vi "USBGetBuffer.vi"() -> ()   [LabVIEW 2012]
uses:
  <vilib>/Instr/_visa.llb/VISA Open Access Mode.ctl
panel:
  out "read buffer 2":string
  out "string":string
  out "16bit integer 2":i16
  out "16bit integer":i16
  out "unsigned 16bit integer 2":u16
  out "unsigned 16bit integer":u16
  out "error out 2":errorcluster
  in  "Access Mode":T1 items=["VISA Defaults"=0, "Exclusive Lock"=1, "Load Configured Settings"=4]
  in  "length (0)":u16
  out "error out":errorcluster
  in  "VISA resource name":refnum<visa-resource-name>
  in  "Request":string="06"
  in  "RequestType":string="80"
  in  "Value":string="0301"
  in  "Index":string="0409"
  out "read buffer":u8[](array[numeric])
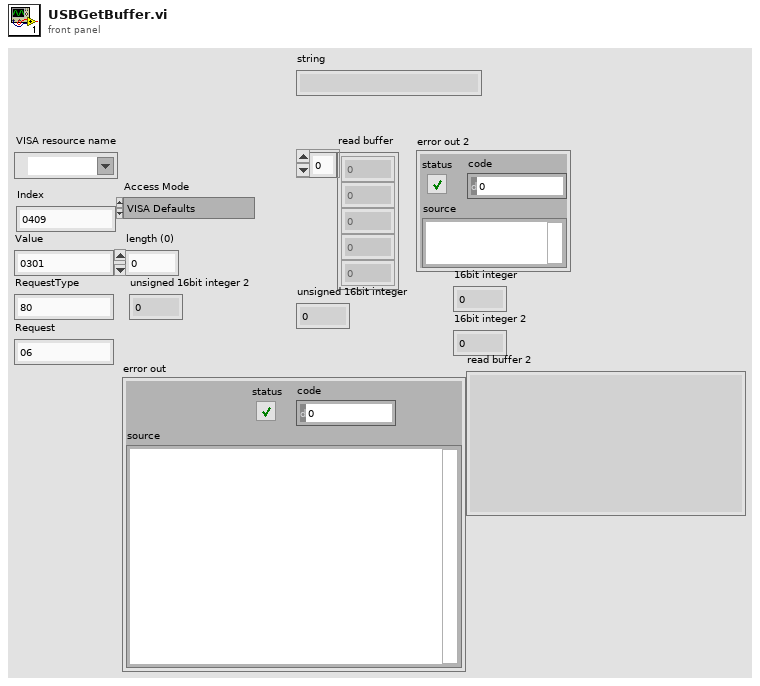
[diagram p1: front panel]
types:
  T1 = typedef "VISA Open Access Mode.ctl" = u32
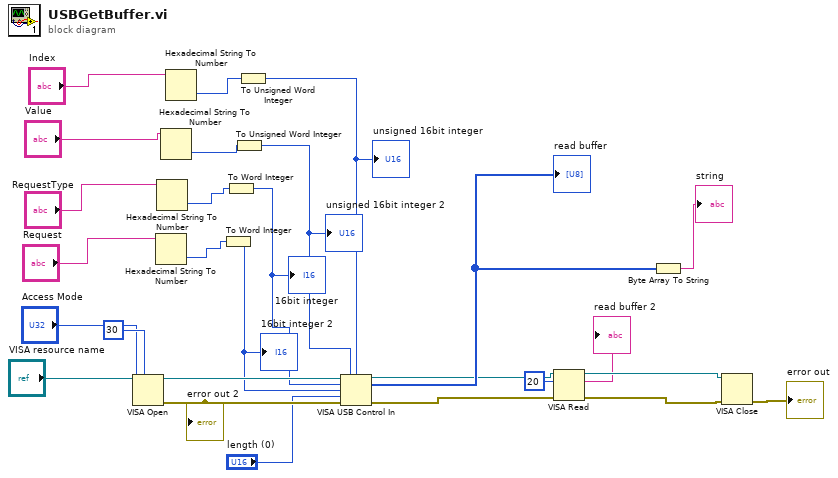
[diagram p0: block diagram]
diagram:
  n1 = VISA Open(timeout (0)=u32 30 ("VISA Open timeout (0)"), access mode="Access Mode", VISA resource name="VISA resource name") -> (VISA resource name=w27:refnum<visa-resource-name>, error out=w26:errorcluster)  [unwired: 2 in]
  "error out 2" <- w26
  n2 = Hexadecimal String To Number(string="Request") -> (number=w9:u32)  [unwired: 2 in, 1 out]
  n3 = Hexadecimal String To Number(string="RequestType") -> (number=w10:u32)  [unwired: 2 in, 1 out]
  n4 = Hexadecimal String To Number(string="Value") -> (number=w11:u32)  [unwired: 2 in, 1 out]
  n5 = Hexadecimal String To Number(string="Index") -> (number=w12:u32)  [unwired: 2 in, 1 out]
  n6 = To Word Integer(number=w9) -> (16bit integer=w18:i16)
  "16bit integer 2" <- w18
  n7 = To Word Integer(number=w10) -> (16bit integer=w19:i16)
  "16bit integer" <- w19
  n8 = To Unsigned Word Integer(number=w11) -> (unsigned 16bit integer=w20:u16)
  "unsigned 16bit integer 2" <- w20
  n9 = To Unsigned Word Integer(number=w12) -> (unsigned 16bit integer=w24:u16)
  "unsigned 16bit integer" <- w24
  n10 = VISA USB Control In(0:w27, 1:w20, 2:w24, 5:w19, 7:w18, 9:"length (0)", 11:w26) -> (4:w6:refnum<visa-resource-name>, 6:w8:u8[], 15:w5:errorcluster)
  "read buffer" <- w8
  n11 = VISA Read(VISA resource name=w6, byte count=u32 20, error in (no error)=w5) -> (VISA resource name out=w4:refnum<visa-resource-name>, read buffer=→"read buffer 2":string, error out=w3:errorcluster)  [unwired: 1 out]
  n12 = Byte Array To String(unsigned byte array=w8) -> (string=→"string":string)
  n13 = VISA Close(VISA resource name=w4, error in (no error)=w3) -> (error out=→"error out":errorcluster)
